vi "sv_Coefficients for Exponential Averaging.vi"(2 "sampling frequency [Hz]":dbl=10000.0 format="%.2f", 3 "time constant [ms]":dbl=125.0 min=0.0 format="%.2f", 4 "exponential mode":enum16{"Slow", "Fast", "Impulse", "Custom"}(ring)=enum."Fast") -> (0 "actual time constant [ms]":dbl=125.0 format="%.2f", 1 "filter coefficients":T1 {"Forward Coefficients" format="%.2f"; "Reverse Coefficients" format="%.2f"})   [LabVIEW 2017]
doc: "Generates the filter coefficients that correspond to the selected exponential mode or custom time constant."
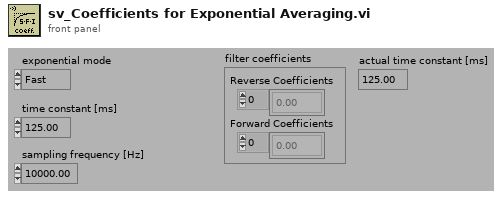
[diagram p1: front panel]
types:
  T1 = cluster{"Reverse Coefficients":dbl[], "Forward Coefficients":dbl[]}
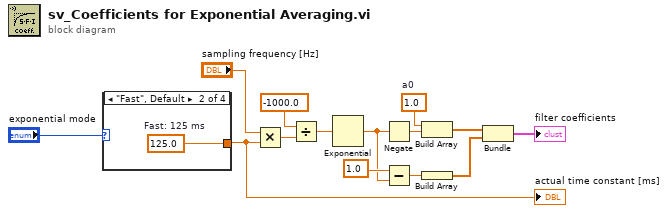
[diagram p0: block diagram]
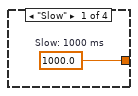
[diagram p2: hidden frame]
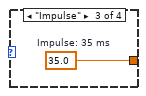
[diagram p3: hidden frame]
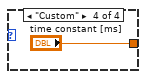
[diagram p4: hidden frame]
diagram:
  w10 = 1.0  # a0
  n1 = case shown="\"Fast\", Default" "exponential mode" {
    tunnel: [w15 w16 w17 "time constant [ms]"] -> w4
    frame "Slow" {
      w15 = 1000.0  # Slow: 1000 ms
    }
    frame "Fast", Default {
      w16 = 125.0  # Fast: 125 ms
    }
    frame "Impulse" {
      w17 = 35.0  # Impulse: 35 ms
    }
    frame "Custom" {
    }
  }
  "actual time constant [ms]" <- w4
  n2 = Multiply(x="sampling frequency [Hz]", y=w4) -> (x*y=w11:dbl)
  n3 = Divide(x=-1000.0, y=w11) -> (x/y=w13:dbl)
  n4 = Exponential(1:w13) -> (0:w8:dbl)
  n5 = Negate(x=w8) -> (-x=w9:dbl)
  n6 = Subtract(x=1.0, y=w8) -> (x-y=w7:dbl)
  n7 = Build Array(w10, w9) -> (w3:dbl[])
  n8 = Build Array(w7) -> (w2:dbl[])
  n9 = Bundle(w3, w2) -> (→"filter coefficients":cluster{dbl[], dbl[]})  [unwired: 1 in]
